vi "DrawMaze.vi"(8 "error in (no error)":errorcluster, 11 "Maze*":refnum<data-value>) -> (0 "error out":errorcluster, 2 "new picture":picture)   [LabVIEW 2016, in "Maze.lvclass"]
uses:
  Maze.lvclass
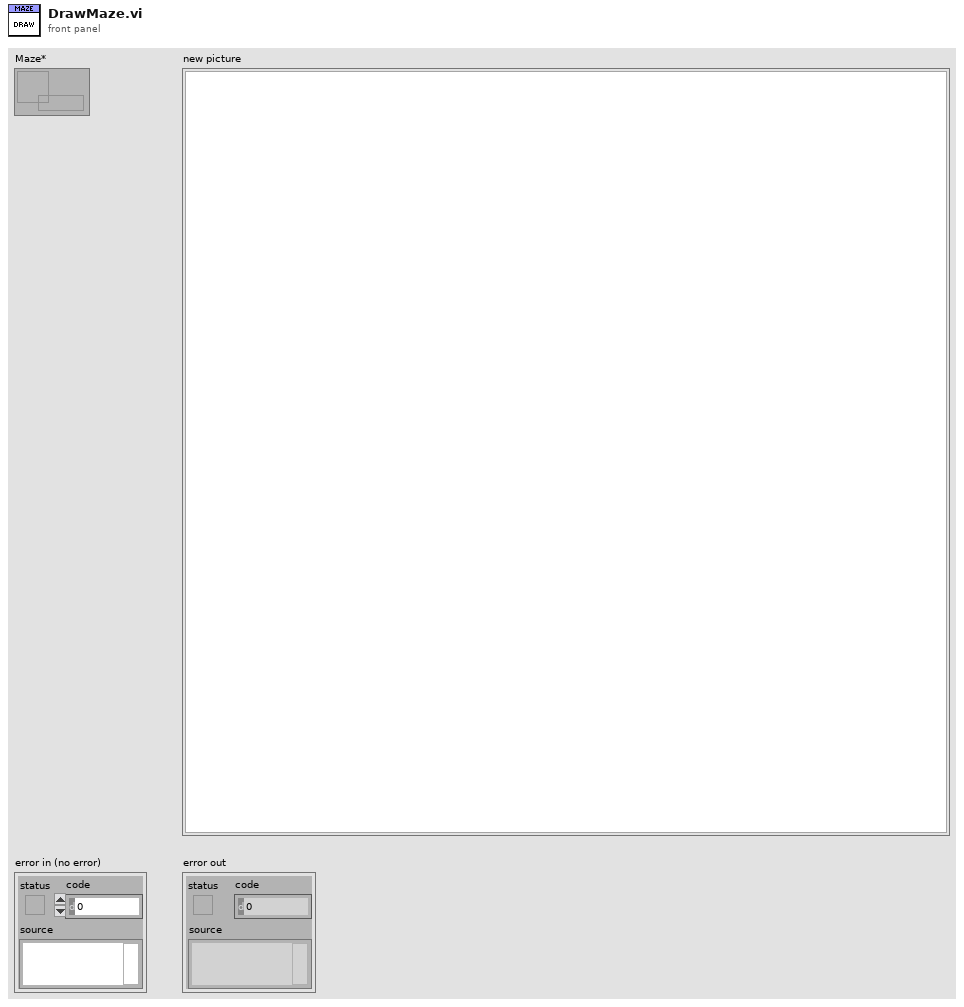
[diagram p1: front panel]
types:
  T1 = typedef "imagedata.ctl" = cluster{"image type":i32, "image depth":i32, "image":u8[], "mask":u8[], "colors":u32[], "Rectangle":cluster{"left":i16, "top":i16, "right":i16, "bottom":i16}}
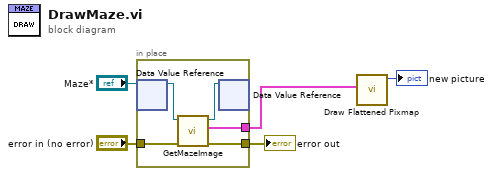
[diagram p0: block diagram]
diagram:
  n1 = in-place {
    in-place-border: [w8] -> w2
    in-place-border: "error in (no error)" -> [w7]
    in-place-border: [w6] -> w3
    n2 = in-place-dvr #1("Maze*") -> (w10:refnum<class "Maze.lvclass">)  [unwired: 1 out]
    n3 = call-dynamic "GetMazeImage.vi"("error in (no error)"=w7, "Maze in"=w10) -> ("error out"=w6:errorcluster, "image data"=w8:T1, "Maze out"=w9:refnum<class "Maze.lvclass">)  [unwired: 7 in]
    n4 = in-place-dvr #1(w9) -> ()  [unwired: 2 out]
  }
  "error out" <- w3
  n5 = call <vilib>:"Draw Flattened Pixmap.vi"("image data"=w2) -> ("new picture"=→"new picture":picture)  [unwired: 8 in]
